vi "CRYASIOTestDriverPresent.vi"(9 "Driver Name":string, 11 "error in (no error)":errorcluster) -> (0 "bResult":bool, 3 "error out":errorcluster)   [LabVIEW 2013]
uses:
  CRY_ASIO.dll
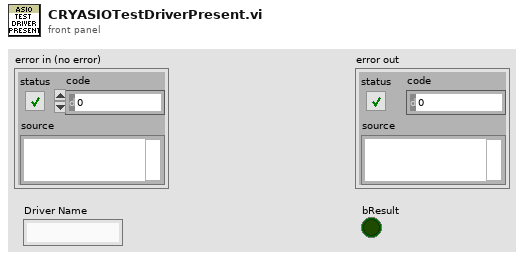
[diagram p1: front panel]
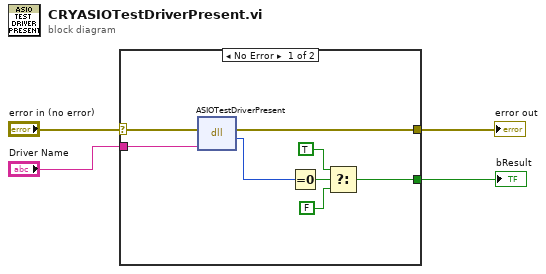
[diagram p0: block diagram]
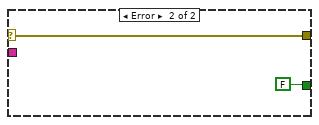
[diagram p2: hidden frame]
diagram:
  n1 = case shown="No Error" "error in (no error)" {
    selector: "error in (no error)" -> [w12 w14]
    tunnel: [w11 w14] -> w3
    tunnel: "Driver Name" -> [w10 _]
    tunnel: [w5 FALSE] -> w1
    frame No Error {
      n2 = dll-call lib="D:/LabView_Project/CRY6181/CRY_ASIO.dll" fn="ASIOTestDriverPresent"(error in=w12, "arg1"=w10) -> (error out=w11:errorcluster, "return type"=w8:i32)  [unwired: 3 in, 1 out]
      n3 = Equal To 0?(x=w8) -> (x = 0?=w9:bool)
      n4 = Select(t=TRUE, s=w9, f=FALSE) -> (s? t:f=w5:bool)
    }
    frame Error {
    }
  }
  "error out" <- w3
  "bResult" <- w1
